vi "Read Project File.vi"(8 "Error In":errorcluster, 11 "path to XML document":path caption="Project File Path") -> (0 "Error Out":errorcluster, 1 "Valid?":bool, 2 "Project Version out":string)   [LabVIEW 2015, in "LV Project Version Check.lvlib"]
uses:
  LV Project Version Check.lvlib
  <vilib>/xml/Load XML File.vi
  <vilib>/xml/Close Reference(Node).vi
  <resource>/objmgr/DOMUserDefRef.rc
  <vilib>/xml/NI_XML.lvlib
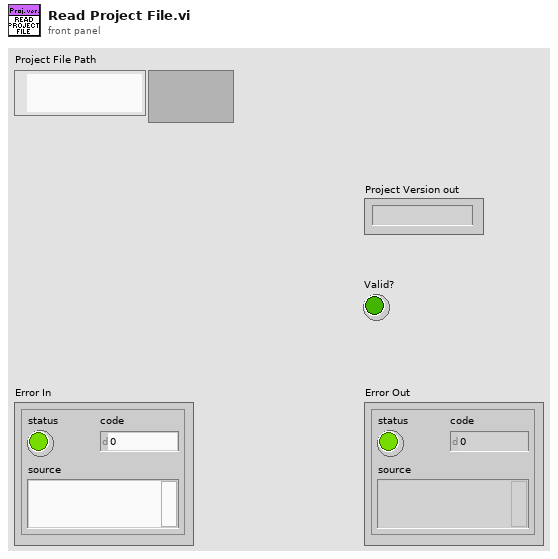
[diagram p1: front panel]
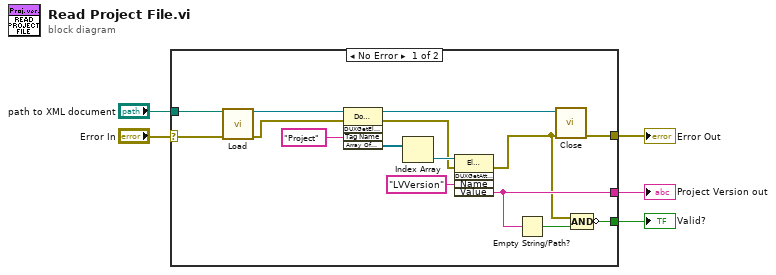
[diagram p0: block diagram]
diagram:
  n1 = case shown="No Error" "Error In" {
    selector: "Error In" -> [w11 w21]
    tunnel: "path to XML document" -> [w18 _]
    tunnel: [w9 _] -> w4
    tunnel: [w10 w21] -> w2
    tunnel: [w6 _] -> w1
    frame No Error {
      n2 = call-poly <vilib>:"Load.vi"("path to XML document"=w18, "error in (no error)"=w11) -> ("DOM document out"=w19:refnum<k20>, "error out"=w17:errorcluster)  [unwired: 11 in, 1 out]
      n3 = invoke class="Document" method="DUXGetElementsByTagName"(reference=w19, error in=w17, "Tag Name"="Project") -> (reference out=w16:refnum<k20>, error out=w12:errorcluster, "Array Of Elements"=w15:refnum<k20>[])  [unwired: 2 in, 2 out]
      n4 = Index Array(array=w15) -> (element=w14:refnum<k20>)  [unwired: 1 in]
      n5 = invoke on="Invoke Node" class="Element" method="DUXGetAttribute"(reference=w14, error in=w12, "Name"="LVVersion") -> (error out=w7:errorcluster, "Value"=w9:string)  [unwired: 2 in, 3 out]
      n6 = Empty String/Path?(string/path=w9) -> (empty?=w8:bool)
      n7 = call-poly <vilib>:"Close.vi"("error in (no error)"=w7, "node"=w16) -> ("error out"=w10:errorcluster)  [unwired: 7 in]
      n8 = Compound Arithmetic op=AND(w7, w8) -> (invert w6:bool)
    }
    frame Error {
    }
  }
  "Error Out" <- w2
  "Project Version out" <- w4
  "Valid?" <- w1
